vi "Control Screen.vi"() -> ()   [LabVIEW 2016]
uses:
  <vilib>/userdefined/High Color/IMAQdx.ctl
  <vilib>/Utility/file.llb/Read From Spreadsheet File (string).vi
  <vilib>/Utility/file.llb/Write To Spreadsheet File (string).vi
  Library_alfa.lvlib
  <vilib>/vision/driver/NI_Vision_Acquisition_Software.lvlib
  <vilib>/vision/NI_Vision_Development_Module.lvlib
panel:
  in  "Сохранить настройки":bool
  out "индикация видео":T1(plugin-control)
  in  "Область измерения":T2 {"Rotation" format="%.2f"; "Left" scale=0.0..1024.0; "Right" scale=0.0..1280.0}
  in  "Параметры измерения":T3={"Contrast"=40, "Filter width"=4, "Steepness"=2, "Subsampling Ratio"=5, "Show Search Area"=FALSE, "Show Search Lines"=FALSE, "Show Edges Found"=FALSE, "Show Result"=TRUE}
  out "16bit integer":i16
  in  "Уровень бинаризации":T4={"Нижний предел"=128.0, "Верхний предел"=255.0} {"Верхний предел" format="%.2f"; "Нижний предел" format="%.2f"}
  in  "A2":dbl
  in  "A1":dbl
  in  "sp_rol_speed":dbl
  in  "vac":dbl
  out "Номер электрода":string caption="EL NUM"
  out "давл в рессив":string caption="PoR (bar)"
  out "Т газа забор":string caption="ToC (C°)"
  out "WRG":string caption="VoC(torr)"
  out "Давление в камере":string caption="PoC(bar)"
  out "T газа в ролик":string caption="TRG (C°)"
  out "давл блок прив":string caption="PRG (bar)"
  out "T ролик (C°)":string caption="TRB (C°)"
  out "Ист вкл инд":bool caption="WORK"
  out "Давление в плазматроне":string caption="PPG (bar)"
  out "T газ (C°)":string caption="TPG (C°)"
  out "Компрессора диод":bool caption="WORK"
  in  "Компрессора выключить":bool
  in  "Компрессора включить":bool
  out "охлаждение инд":bool caption="WORK"
  in  "Охлаждение выкл":bool
  in  "Охлаждение вкл":bool
  in  "КЗ СТОП":bool
  out "Бункер закрыт":bool caption="WORK"
  in  "Закрыть бункер кн":bool
  in  "Открыть бункер кн":bool
  out "Индикатор положения полки":string
  in  "Бункер на след полку кн":bool
  in  "Аварийный стоп":bool
  in  "Автозапуск регулятора кн":bool
  out "Индикатор автозапуска регулятора":bool
  out "Максимальная подача":string caption="MAX SPEED"
  out "Текущая подача":string caption="SPEED"
  out "Текущий зазор":string caption="DISTANS"
  out "Задание зазора":string caption="SET DISTANS"
  in  "Пересыпное в бол кн":bool
  in  "Пересыпное в малый кн":bool
  out "Пересыпное большой":bool caption="WORK"
  out "Пересыпное малый":bool caption="LOAD"
  out "Бараб V":dbl(knob) caption="ROLLER SPEED" scale=0.0..24000.0
  out "V pl":dbl(knob) caption="VOLTAGE" scale=0.0..100.0
  out "Ток плазматрона":dbl(knob) caption="CURRENT" scale=0.0..2000.0
  out "V бараб":string caption="ROLLER"
  out "Задание част вращ барабанов":string caption="ROLLER SPEED"
  out "вибро 1":string caption="V1 (mm\\s)"
  out "вибро 2":string caption="V1 (mm\\s)"
  out "Ток барабана 2":string caption="S2(A)"
  out "Ток барабана 1":string caption="S1(A)"
  in  "Толкатель поз 2":i32 format="%x"
  in  "Плаз поз 2":i32 format="%x"
  out "плазма рабочее":bool caption="WORK"
  out "положение толк мм":string caption="mm"
  out "Положение плазматрона":string caption="mm"
  out "плазма от заг":bool caption="WORK"
  out "плазма к заг":bool caption="LOAD"
  in  "плазма назад кн":bool
  in  "плазма в раб кн":bool
  out "Толкатель в крайнем":bool caption="WORK"
  out "v_tol":string caption="V (mm\\min)"
  out "v_pl":string caption="V (mm\\min)"
  out "Пол плазматрона":dbl(slide)
  out "Пол толк":dbl(slide) scale=0.0..100.0
  out "Толкатель в рабочем диод":bool caption="WORK"
  out "Толкатель под загрузку диод":bool caption="LOAD"
  in  "Толкатель в рабочее кн":bool
  in  "Толкатель под загрузку кн":bool
  in  "v_pl":i32 format="%x"
  in  "v_tol":i32 format="%x"
  in  "дат вибр 2":i32 format="%x"
  in  "дат вибр1":i32 format="%x"
  in  "ОШИБКА":i32 format="%x"
  in  "T газа в ролик":i32 format="%x"
  in  "давл блок прив":dbl
  in  "Т газа забор":i32 format="%x"
  in  "давл в рессив":dbl
  out "T4 (C°)":string caption="TB2.2 (C°)"
  out "T3 (C°)":string caption="TB2.1 (C°)"
  out "T2 (C°)":string caption="TB1.2 (C°)"
  out "T1 (C°)":string caption="TB1.1 (C°)"
  in  "Подача":i32 format="%x"
  in  "PV":i32 format="%x"
  in  "Roll speed":i32 format="%x"
  in  "P C1":i32 format="%x"
  in  "P plaz":dbl
  in  "ROLLER Speed":dbl
  in  "V плазматр":i32 format="%x"
  in  "Толкатель поз":i32 format="%x"
  in  "Плаз поз":i32 format="%x"
  in  "А плазм":i32 format="%x"
  in  "T GAS":i32 format="%x"
  in  "T ROLLER":i32 format="%x"
  in  "T4":dbl
  in  "T3":i32 format="%x"
  in  "T2":i32 format="%x"
  in  "T1":dbl
  out "Выход":bool caption="WORK"
  in  "Архив":bool
  in  "Газовая система":bool
  in  "Вакуумная система":bool
  in  "Выход":bool
  out "Текущее время":string
  # "DISPENSER"
  # "GAS SYSTEM"
  # "COOLING SYSTEM"
  # "ELECTRODS STORE"
  # "PERFORMANCE PARAMETERS"
  # "PULLEYS"
  # "SP FEED"
  # "PL FEED"
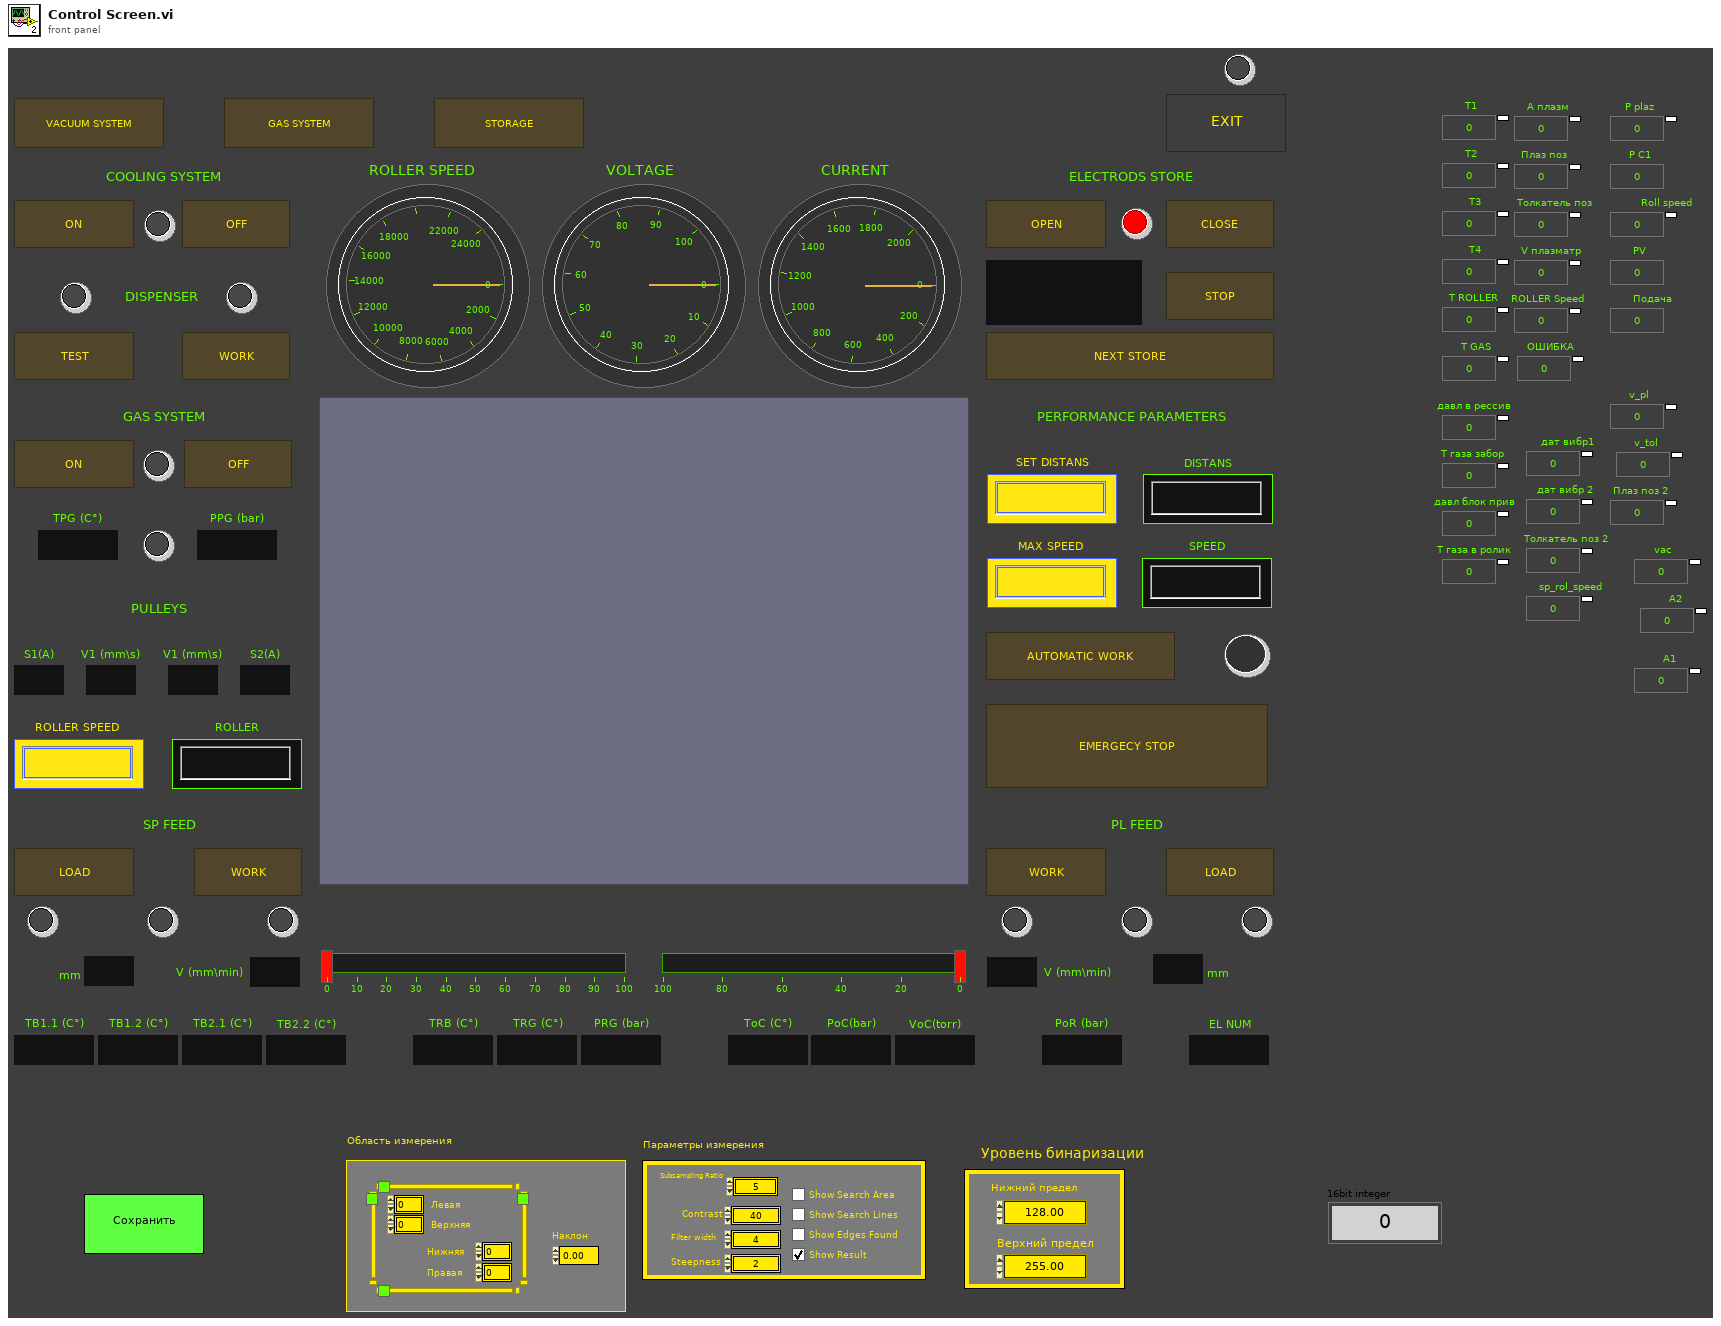
[diagram p1: front panel]
types:
  T1 = typedef "IMAQ Image.ctl" = refnum<image>
  T2 = typedef "IMAQ Rectangle" = cluster{"Left":i32, "Top":i32, "Right":i32, "Bottom":i32, "Rotation":dbl}
  T3 = cluster{"Contrast":i32, "Filter width":i32, "Steepness":i32, "Subsampling Ratio":u32, "Show Search Area":bool, "Show Search Lines":bool, "Show Edges Found":bool, "Show Result":bool}
  T4 = cluster{"Нижний предел":sgl, "Верхний предел":sgl}
  T5 = typedef "Library_alfa.lvlib/IMAQdx.ctl" = refnum<k21>
  T6 = enum16{"open", "replace", "create", "open or create", "replace or create", "replace or create with confirmation"}
  T7 = typedef "Image Type" = u32
  T8 = cluster{i32, i32, i32, u32, "Boolean":bool, "Boolean":bool, "Boolean":bool, "Boolean":bool}
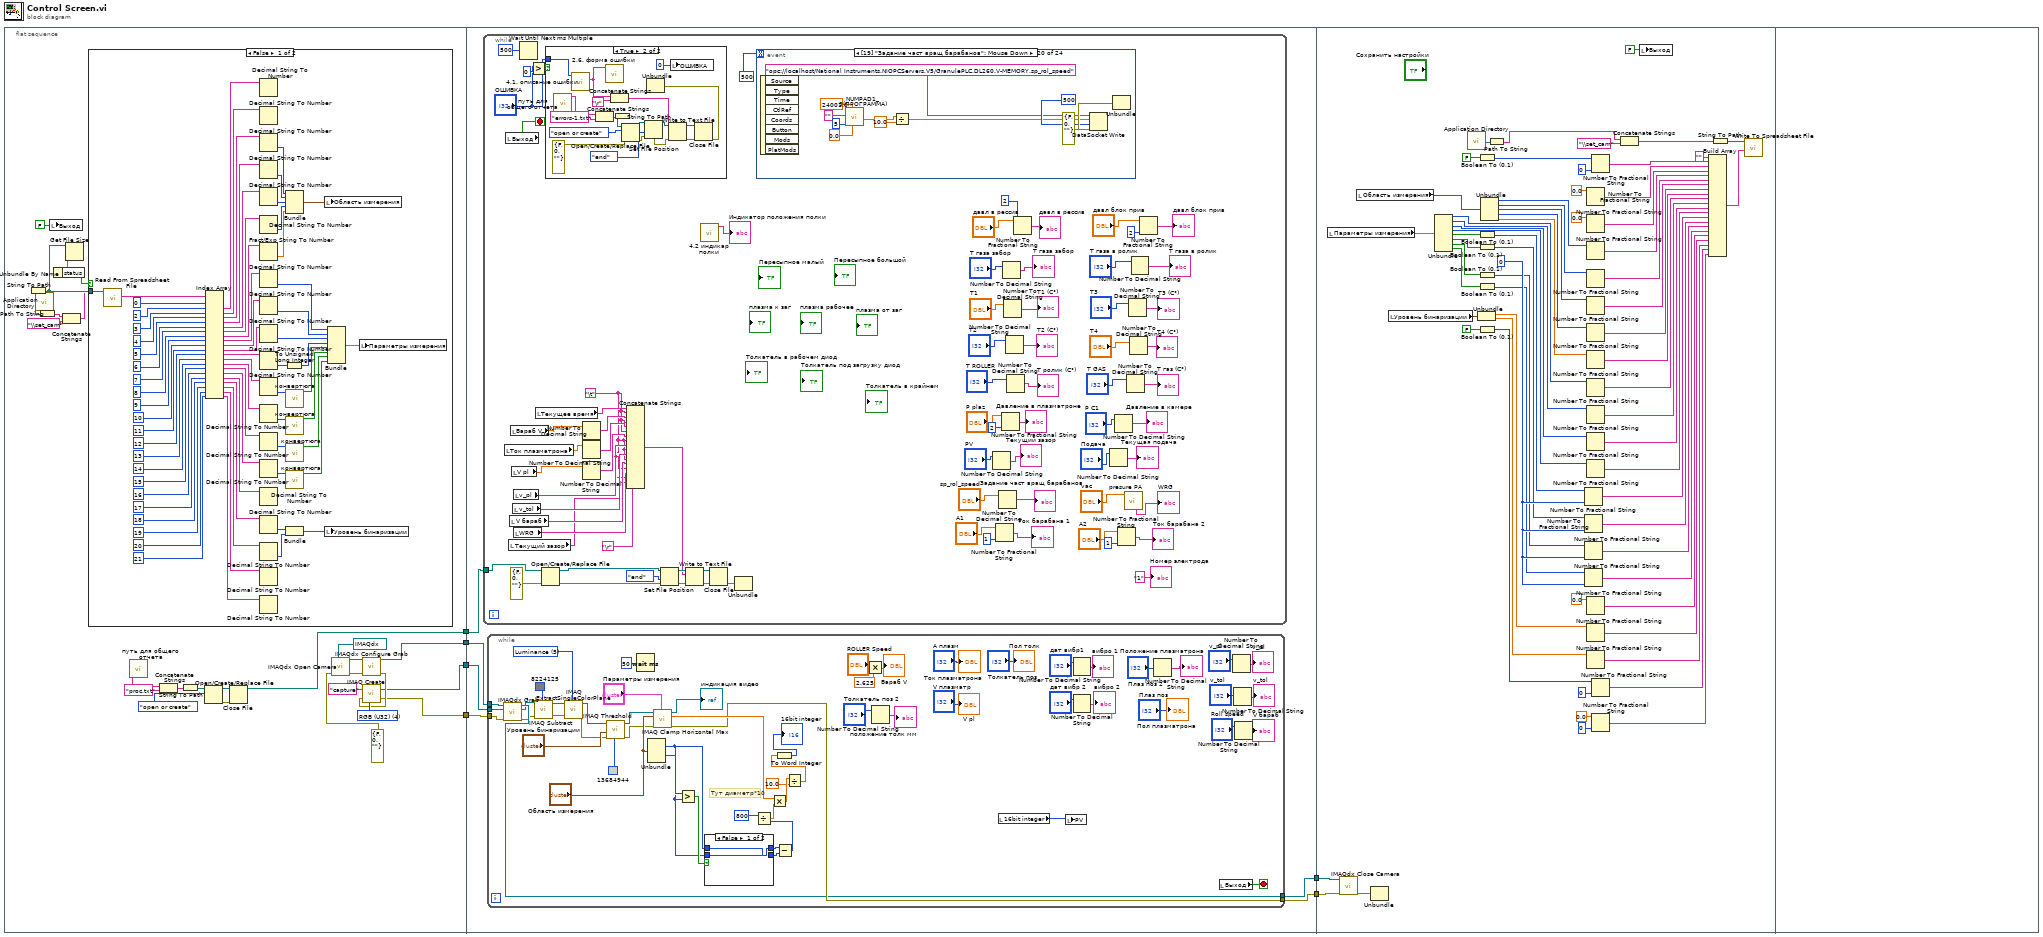
[diagram p0: block diagram]
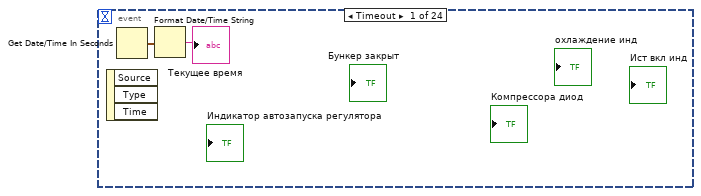
[diagram p5: hidden frame]
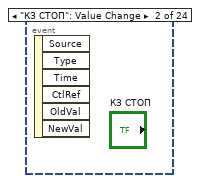
[diagram p6: hidden frame]
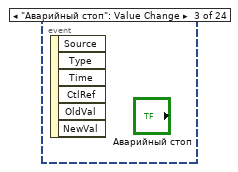
[diagram p7: hidden frame]
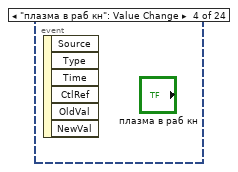
[diagram p8: hidden frame]
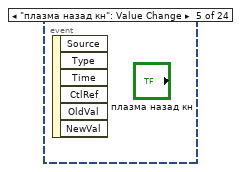
[diagram p9: hidden frame]
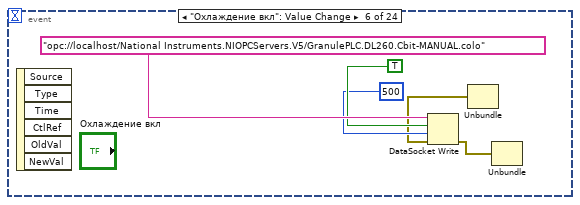
[diagram p10: hidden frame]
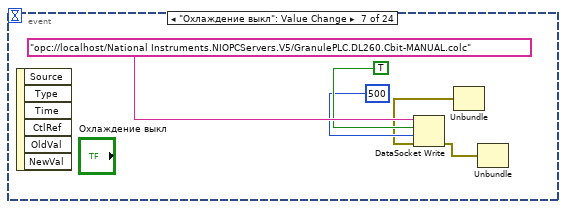
[diagram p11: hidden frame]
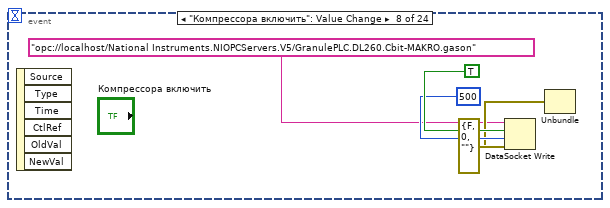
[diagram p12: hidden frame]
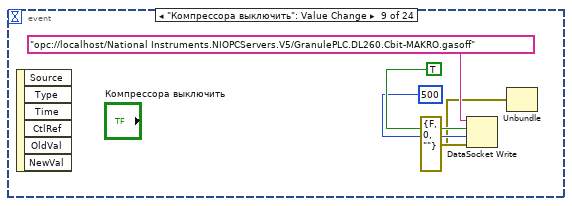
[diagram p13: hidden frame]
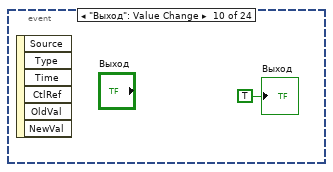
[diagram p14: hidden frame]
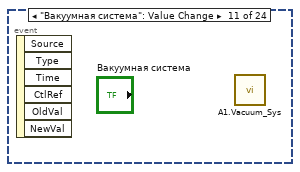
[diagram p15: hidden frame]
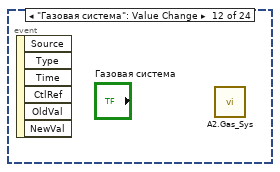
[diagram p16: hidden frame]
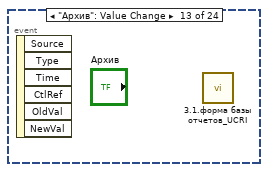
[diagram p17: hidden frame]
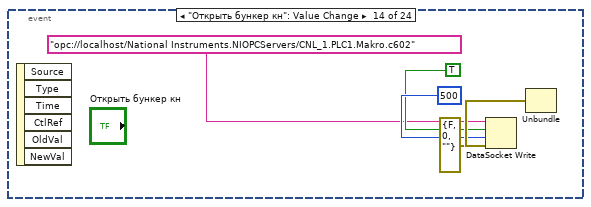
[diagram p18: hidden frame]
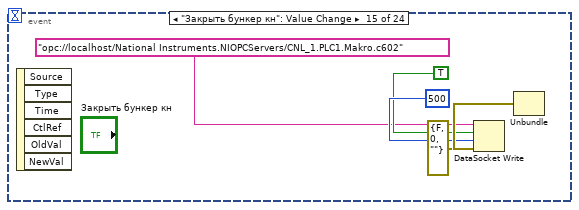
[diagram p19: hidden frame]
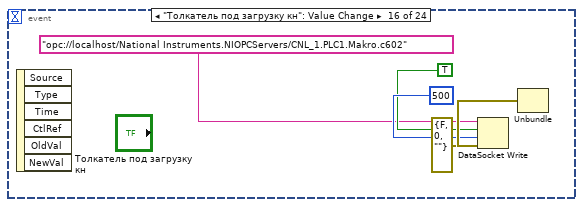
[diagram p20: hidden frame]
diagram:
  n1 = flat-sequence {
    tunnel: [w10] -> w4
    tunnel: [w9] -> w3
    tunnel: [w8] -> w2
    tunnel: [w7] -> w1
    tunnel: [w104] -> w6
    tunnel: [w103] -> w5
    tunnel: w4 -> [w102]
    tunnel: w3 -> [w101]
    tunnel: w2 -> [w100]
    tunnel: w1 -> [w99]
    tunnel: w6 -> [w405]
    tunnel: w5 -> [w404]
    frame #0 {
      w14 = T7 4 items=["Grayscale (U8)", "Grayscale (I16)", "Grayscale (SGL)", "Complex (CSG)", "RGB (U32)", "HSL (U32)", "RGB (U64)", "Grayscale (U16)"] ("Image Type")
      n2 = call <vilib>:"Application Directory.vi"() -> ("Application Directory"=w18:path)
      n3 = Path To String(path=w18) -> (string=w19:string)
      n4 = local write "Выход"(FALSE ("Выход")) -> ()
      n5 = Concatenate Strings(w19, "\\set_cam" ("string")) -> (w21:string)
      n6 = String To Path(string=w21) -> (path=w24:path)
      n7 = Get File Size(file=w24) -> (0:w22:errorcluster)  [unwired: 1 in, 2 out]
      n8 = Unbundle By Name(w22) -> ("status"=w23:bool)
      n9 = case shown="False" w23 {
        tunnel: w24 -> [w98 _]
        frame False {
          n10 = call-poly <vilib>:"Read From Spreadsheet File.vi"("file path (dialog if empty)"=w98) -> ("first row"=w97:string[])  [unwired: 6 in, 4 out]
          n11 = Index Array(array=w97, index #1=0 ("index"), index #2=2 ("index"), index #3=3 ("index"), index #4=4 ("index"), index #5=5 ("index"), index #6=6 ("index"), index #7=7 ("index"), index #8=8 ("index"), index #9=9 ("index"), index #10=10 ("index"), index #11=11 ("index"), index #12=12 ("index"), index #13=13 ("index"), index #14=14 ("index"), index #15=15 ("index"), index #16=16 ("index"), index #17=17 ("index"), index #18=18 ("index"), index #19=19 ("index"), index #20=20 ("index"), index #21=21 ("index")) -> (element #2=w94:string, element #3=w92:string, element #4=w85:string, element #5=w83:string, element #6=w81:string, element #7=w79:string, element #8=w77:string, element #9=w68:string, element #10=w66:string, element #11=w64:string, element #12=w62:string, element #13=w60:string, element #14=w58:string, element #15=w56:string, element #16=w54:string, element #17=w44:string, element #18=w40:string, element #19=w38:string, element #20=w36:string, element #21=w33:string)  [unwired: 1 out]
          n12 = Decimal String To Number(string=w94) -> ()  [unwired: 2 in, 2 out]
          n13 = Decimal String To Number(string=w92) -> ()  [unwired: 2 in, 2 out]
          n14 = Decimal String To Number(string=w85) -> (number=w90:i32)  [unwired: 2 in, 1 out]
          n15 = Decimal String To Number(string=w83) -> (number=w89:i32)  [unwired: 2 in, 1 out]
          n16 = Decimal String To Number(string=w81) -> (number=w88:i32)  [unwired: 2 in, 1 out]
          n17 = Decimal String To Number(string=w79) -> (number=w87:i32)  [unwired: 2 in, 1 out]
          n18 = Fract/Exp String To Number(string=w77) -> (number=w76:dbl)  [unwired: 3 in, 1 out]
          n19 = Decimal String To Number(string=w68) -> (number=w74:i32)  [unwired: 2 in, 1 out]
          n20 = Decimal String To Number(string=w66) -> (number=w73:i32)  [unwired: 2 in, 1 out]
          n21 = Decimal String To Number(string=w64) -> (number=w72:i32)  [unwired: 2 in, 1 out]
          n22 = Decimal String To Number(string=w62) -> (number=w71:i32)  [unwired: 2 in, 1 out]
          n23 = Decimal String To Number(string=w60) -> (number=w53:i32)  [unwired: 2 in, 1 out]
          n24 = Decimal String To Number(string=w58) -> (number=w51:i32)  [unwired: 2 in, 1 out]
          n25 = Decimal String To Number(string=w56) -> (number=w49:i32)  [unwired: 2 in, 1 out]
          n26 = Decimal String To Number(string=w54) -> (number=w47:i32)  [unwired: 2 in, 1 out]
          n27 = Decimal String To Number(string=w44) -> ()  [unwired: 2 in, 2 out]
          n28 = Decimal String To Number(string=w40) -> (number=w39:i32)  [unwired: 2 in, 1 out]
          n29 = Decimal String To Number(string=w38) -> (number=w37:i32)  [unwired: 2 in, 1 out]
          n30 = Decimal String To Number(string=w36) -> ()  [unwired: 2 in, 2 out]
          n31 = Decimal String To Number(string=w33) -> ()  [unwired: 2 in, 2 out]
          n32 = To Unsigned Long Integer(number=w71) -> (unsigned 32bit integer=w70:u32)
          n33 = Bundle(w90, w89, w88, w87, w76) -> (w91:cluster{i32, i32, i32, i32, dbl})  [unwired: 1 in]
          n34 = call "конвертюга.vi"("Numeric"=w53) -> ("Boolean"=w52:bool)  [unwired: 10 in]
          n35 = call "конвертюга.vi"("Numeric"=w51) -> ("Boolean"=w50:bool)  [unwired: 10 in]
          n36 = call "конвертюга.vi"("Numeric"=w49) -> ("Boolean"=w48:bool)  [unwired: 10 in]
          n37 = call "конвертюга.vi"("Numeric"=w47) -> ("Boolean"=w46:bool)  [unwired: 10 in]
          n38 = Bundle(w39, w37) -> (w43:cluster{i32, i32})  [unwired: 1 in]
          n39 = local write "Область измерения"(w91) -> ()
          n40 = local write "Уровень бинаризации"(w43) -> ()
          n41 = Bundle(w74, w73, w72, w70, "Boolean"=w52, "Boolean"=w50, "Boolean"=w48, "Boolean"=w46) -> (w75:T8)  [unwired: 1 in]
          n42 = local write "Параметры измерения"(w75) -> ()
        }
        frame True {
        }
      }
      n43 = call "путь для общего отчета.vi"() -> ("path_out 2"=w28:string)  [unwired: 11 in]
      n44 = Concatenate Strings(w28, "proc.txt") -> (w26:string)
      n45 = String To Path(string=w26) -> (path=w29:path)
      n46 = Open/Create/Replace File(file path (use dialog)=w29, operation (0:open)=T6."open or create") -> (refnum out=w32:refnum<file>, error out=w31:errorcluster)  [unwired: 4 in, 1 out]
      n47 = Close File(refnum=w32, error in=w31) -> (path=w7:path)  [unwired: 1 out]
      n48 = call <vilib>:"IMAQdx Open Camera.vi"("error in"=errorcluster {"status"=FALSE, "code"=0, "source"=""}, "Session In"=T5 "cam3") -> ("error out"=w15:errorcluster, "Session Out"=w12:T5)  [unwired: 8 in]
      n49 = call <vilib>:"IMAQdx Configure Grab.vi"("error in"=w15, "Session In"=w12) -> ("error out"=w11:errorcluster, "Session Out"=w8:T5)  [unwired: 8 in]
      n50 = call "IMAQ Create"("Image Name"="capture", "Image Type"=w14, "error in (no error)"=w11) -> ("New Image"=w10:T1, "error out"=w9:errorcluster)  [unwired: 2 in]
    }
    frame #1 {
      n51 = while {
        tunnel: w99 -> [w181]
        stop <- w237 stop-if-true
        w169 = "\t"
        n52 = local read "Ток плазматрона"() -> (w179:dbl)
        n53 = local read "Выход"() -> (w237:bool)
        n54 = local read "Текущий зазор"() -> (w168:string)
        n55 = local read "V бараб"() -> (w171:string)
        n56 = local read "Бараб V"() -> (w180:dbl)
        n57 = local read "V pl"() -> (w178:dbl)
        n58 = local read "v_tol"() -> (w172:string)
        n59 = local read "v_pl"() -> (w173:string)
        n60 = local read "WRG"() -> (w170:string)
        n61 = Wait Until Next ms Multiple(millisecond multiple=u32 500) -> ()  [unwired: 1 out]
        n62 = Greater?(x="ОШИБКА", y=i16 0) -> (0:w224:bool)
        n63 = local read "Текущее время"() -> (w177:string)
        n64 = Open/Create/Replace File(file path (use dialog)=w181, error in=errorcluster {"status"=FALSE, "code"=0, "source"=""}) -> (refnum out=w190:refnum<file>, error out=w188:errorcluster)  [unwired: 4 in, 1 out]
        n65 = case shown="True" w224 {
          tunnel: "ОШИБКА" -> [_ w241]
          frame False {
          }
          frame True {
            n66 = call "путь для общего отчета.vi"() -> ("path_out 2"=w242:string)  [unwired: 11 in]
            n67 = call "4.1. описание ошибки.vi"("Numeric"=w241) -> ("Полностью"=w240:string)  [unwired: 8 in, 2 out]
            n68 = Concatenate Strings(w242, "errors-1.txt") -> (w256:string)
            n69 = call "2.6. форма ошибки.vi"("Описание ошибки"=w240) -> ()  [unwired: 11 in]
            n70 = Concatenate Strings(w240, "\r") -> (w244:string)
            n71 = String To Path(string=w256) -> (path=w258:path)
            n72 = Open/Create/Replace File(file path (use dialog)=w258, error in=errorcluster {"status"=FALSE, "code"=0, "source"=""}, operation (0:open)=T6."open or create") -> (refnum out=w251:refnum<file>, error out=w253:errorcluster)  [unwired: 3 in, 1 out]
            n73 = Set File Position(refnum=w251, from (0:start)=enum16{"start", "end", "current"}."end", error in=w253) -> (refnum out=w249:refnum<file>, error out=w250:errorcluster)  [unwired: 1 in]
            n74 = Write to Text File(file (use dialog)=w249, text=w244, error in=w250) -> (refnum out=w248:refnum<file>, error out=w247:errorcluster)  [unwired: 1 in, 1 out]
            n75 = local write "ОШИБКА"(i16 0 ("Ошибка1")) -> ()
            n76 = Close File(refnum=w248, error in=w247) -> (error out=w246:errorcluster)  [unwired: 1 out]
            n77 = Unbundle(w246) -> ()  [unwired: 3 out]
          }
        }
        n78 = Number To Decimal String(number=w178) -> (decimal integer string=w174:string)  [unwired: 1 in]
        n79 = Number To Decimal String(number=w180) -> (decimal integer string=w176:string)  [unwired: 1 in]
        n80 = Number To Decimal String(number=w179) -> (decimal integer string=w175:string)  [unwired: 1 in]
        n81 = Concatenate Strings(w177, w169, w176, w169, w175, w169, w174, w169, w173, w169, w172, w169, w171, w169, w170, w169, w168, "\r") -> (w166:string)
        n82 = Set File Position(refnum=w190, from (0:start)=enum16{"start", "end", "current"}."end", error in=w188) -> (refnum out=w187:refnum<file>, error out=w186:errorcluster)  [unwired: 1 in]
        n83 = Write to Text File(file (use dialog)=w187, text=w166, error in=w186) -> (refnum out=w185:refnum<file>, error out=w184:errorcluster)  [unwired: 1 in, 1 out]
        n84 = call "4.2 индикар полки.vi"() -> ("текущее положение"=→"Индикатор положения полки":string)  [unwired: 11 in]
        n85 = Close File(refnum=w185, error in=w184) -> (error out=w183:errorcluster)  [unwired: 1 out]
        n86 = Unbundle(w183) -> ()  [unwired: 3 out]
        n87 = event shown="[19] \"Задание част вращ барабанов\": Mouse Down" {
          selector: _ -> [_ _ _ _ _ _ _ _ _ _ _ _ _ _ _ _ _ _ _ _ _ _ _ _]
          dyn-events: _ -> [_ _ _ _ _ _ _ _ _ _ _ _ _ _ _ _ _ _ _ _ _ _ _ _]
          timeout: 500 -> [_ _ _ _ _ _ _ _ _ _ _ _ _ _ _ _ _ _ _ _ _ _ _ _]
          event Timeout {
            n88 = event-data() -> ()  [unwired: 1 in, 3 out]
            n89 = Get Date/Time In Seconds() -> (seconds since 1Jan1904=w260:timestamp)
            n90 = Format Date/Time String(seconds (now)=w260) -> (date/time string=→"Текущее время":string)  [unwired: 2 in]
          }
          event "КЗ СТОП": Value Change {
            n91 = event-data() -> ()  [unwired: 1 in, 6 out]
          }
          event "Аварийный стоп": Value Change {
            n92 = event-data() -> ()  [unwired: 1 in, 6 out]
          }
          event "плазма в раб кн": Value Change {
            n93 = event-data() -> ()  [unwired: 1 in, 6 out]
          }
          event "плазма назад кн": Value Change {
            n94 = event-data() -> ()  [unwired: 1 in, 6 out]
          }
          event "Охлаждение вкл": Value Change {
            n95 = event-data() -> ()  [unwired: 1 in, 6 out]
            n96 = DataSocket Write(9:500 ("ms timeout (0)"), 10:TRUE, 11:"opc://localhost/National Instruments.NIOPCServers.V5/GranulePLC.DL260.Cbit-MANUAL.colo" ("connection in")) -> (0:w261:errorcluster)  [unwired: 1 in, 2 out]
            n97 = Unbundle(w261) -> ()  [unwired: 3 out]
            n98 = Unbundle(w261) -> ()  [unwired: 3 out]
          }
          event "Охлаждение выкл": Value Change {
            n99 = event-data() -> ()  [unwired: 1 in, 6 out]
            n100 = DataSocket Write(9:500 ("ms timeout (0)"), 10:TRUE, 11:"opc://localhost/National Instruments.NIOPCServers.V5/GranulePLC.DL260.Cbit-MANUAL.colc" ("connection in")) -> (0:w265:errorcluster)  [unwired: 1 in, 2 out]
            n101 = Unbundle(w265) -> ()  [unwired: 3 out]
            n102 = Unbundle(w265) -> ()  [unwired: 3 out]
          }
          event "Компрессора включить": Value Change {
            n103 = event-data() -> ()  [unwired: 1 in, 6 out]
            n104 = DataSocket Write(8:errorcluster {"status"=FALSE, "code"=0, "source"=""} ("error in (no error)"), 9:500 ("ms timeout (0)"), 10:TRUE, 11:"opc://localhost/National Instruments.NIOPCServers.V5/GranulePLC.DL260.Cbit-MAKRO.gason" ("connection in")) -> (0:w270:errorcluster)  [unwired: 2 out]
            n105 = Unbundle(w270) -> ()  [unwired: 3 out]
          }
          event "Компрессора выключить": Value Change {
            n106 = event-data() -> ()  [unwired: 1 in, 6 out]
            n107 = DataSocket Write(8:errorcluster {"status"=FALSE, "code"=0, "source"=""} ("error in (no error)"), 9:500 ("ms timeout (0)"), 10:TRUE, 11:"opc://localhost/National Instruments.NIOPCServers.V5/GranulePLC.DL260.Cbit-MAKRO.gasoff" ("connection in")) -> (0:w274:errorcluster)  [unwired: 2 out]
            n108 = Unbundle(w274) -> ()  [unwired: 3 out]
          }
          event "Выход": Value Change {
            n109 = event-data() -> ()  [unwired: 1 in, 6 out]
            "Выход" <- TRUE ("Выход")
          }
          event "Вакуумная система": Value Change {
            n110 = event-data() -> ()  [unwired: 1 in, 6 out]
            n111 = call "A1.Vacuum_Sys.vi"() -> ()  [unwired: 12 in]
          }
          event "Газовая система": Value Change {
            n112 = event-data() -> ()  [unwired: 1 in, 6 out]
            n113 = call "A2.Gas_Sys.vi"() -> ()  [unwired: 12 in]
          }
          event "Архив": Value Change {
            n114 = event-data() -> ()  [unwired: 1 in, 6 out]
            n115 = call "3.1.форма базы отчетов_UCRI.vi"() -> ()  [unwired: 12 in]
          }
          event "Открыть бункер кн": Value Change {
            n116 = event-data() -> ()  [unwired: 1 in, 6 out]
            n117 = DataSocket Write(8:errorcluster {"status"=FALSE, "code"=0, "source"=""} ("error in (no error)"), 9:500 ("ms timeout (0)"), 10:TRUE, 11:"opc://localhost/National Instruments.NIOPCServers/CNL_1.PLC1.Makro.c602" ("connection in")) -> (0:w284:errorcluster)  [unwired: 2 out]
            n118 = Unbundle(w284) -> ()  [unwired: 3 out]
          }
          event "Закрыть бункер кн": Value Change {
            n119 = event-data() -> ()  [unwired: 1 in, 6 out]
            n120 = DataSocket Write(8:errorcluster {"status"=FALSE, "code"=0, "source"=""} ("error in (no error)"), 9:500 ("ms timeout (0)"), 10:TRUE, 11:"opc://localhost/National Instruments.NIOPCServers/CNL_1.PLC1.Makro.c602" ("connection in")) -> (0:w289:errorcluster)  [unwired: 2 out]
            n121 = Unbundle(w289) -> ()  [unwired: 3 out]
          }
          event "Толкатель под загрузку кн": Value Change {
            n122 = event-data() -> ()  [unwired: 1 in, 6 out]
            n123 = DataSocket Write(8:errorcluster {"status"=FALSE, "code"=0, "source"=""} ("error in (no error)"), 9:500 ("ms timeout (0)"), 10:TRUE, 11:"opc://localhost/National Instruments.NIOPCServers/CNL_1.PLC1.Makro.c602" ("connection in")) -> (0:w294:errorcluster)  [unwired: 2 out]
            n124 = Unbundle(w294) -> ()  [unwired: 3 out]
          }
          event "Толкатель в рабочее кн": Value Change {
            n125 = event-data() -> ()  [unwired: 1 in, 6 out]
            n126 = DataSocket Write(8:errorcluster {"status"=FALSE, "code"=0, "source"=""} ("error in (no error)"), 9:500 ("ms timeout (0)"), 10:TRUE, 11:"opc://localhost/National Instruments.NIOPCServers/CNL_1.PLC1.Makro.c602" ("connection in")) -> (0:w295:errorcluster)  [unwired: 2 out]
            n127 = Unbundle(w295) -> ()  [unwired: 3 out]
          }
          event "Бункер на след полку кн": Value Change {
            n128 = event-data() -> ()  [unwired: 1 in, 6 out]
            n129 = DataSocket Write(8:errorcluster {"status"=FALSE, "code"=0, "source"=""} ("error in (no error)"), 9:500 ("ms timeout (0)"), 10:TRUE, 11:"opc://localhost/National Instruments.NIOPCServers/CNL_1.PLC1.Makro.c602" ("connection in")) -> (0:w304:errorcluster)  [unwired: 2 out]
            n130 = Unbundle(w304) -> ()  [unwired: 3 out]
          }
          event "Автозапуск регулятора кн": Value Change {
            n131 = event-data() -> ()  [unwired: 1 in, 6 out]
            n132 = DataSocket Write(8:errorcluster {"status"=FALSE, "code"=0, "source"=""} ("error in (no error)"), 9:500 ("ms timeout (0)"), 10:TRUE, 11:"opc://localhost/National Instruments.NIOPCServers.V5/GranulePLC.DL260.Cbit-MAKRO.rid_run" ("connection in")) -> (0:w309:errorcluster)  [unwired: 2 out]
            n133 = Unbundle(w309) -> ()  [unwired: 3 out]
          }
          event "Задание част вращ барабанов": Mouse Down {
            n134 = event-data() -> ()  [unwired: 1 in, 8 out]
            n135 = call "NUMPAD1_9(ПРОГРАММА).vi"("МИНИМАЛЬНОЕ ЗНАЧЕНИЕ"=0.0, "МАКСИМАЛЬНОЕ ЗНАЧЕНИЕ"=24001.0, "ДЛИННА СЛОВА"=i8 5, "ТЕКУЩЕЕ ЗНАЧЕНИЕ"="") -> ("exit"=w311:dbl)  [unwired: 6 in, 1 out]
            n136 = Divide(x=w311, y=10.0) -> (x/y=w312:dbl)
            n137 = DataSocket Write(8:errorcluster {"status"=FALSE, "code"=0, "source"=""} ("error in (no error)"), 9:500 ("ms timeout (0)"), 10:w312, 11:"opc://localhost/National Instruments.NIOPCServers.V5/GranulePLC.DL260.V-MEMORY.sp_rol_speed" ("connection in")) -> (0:w320:errorcluster)  [unwired: 2 out]
            n138 = Unbundle(w320) -> ()  [unwired: 3 out]
          }
          event "Максимальная подача": Mouse Down {
            n139 = event-data() -> ()  [unwired: 1 in, 8 out]
            n140 = DataSocket Write(8:errorcluster {"status"=FALSE, "code"=0, "source"=""} ("error in (no error)"), 9:500 ("ms timeout (0)"), 10:TRUE, 11:"opc://localhost/National Instruments.NIOPCServers/CNL_1.PLC1.Makro.c602" ("connection in")) -> (0:w325:errorcluster)  [unwired: 2 out]
            n141 = Unbundle(w325) -> ()  [unwired: 3 out]
          }
          event "Пересыпное в малый кн": Value Change {
            n142 = event-data() -> ()  [unwired: 1 in, 6 out]
            n143 = DataSocket Write(8:errorcluster {"status"=FALSE, "code"=0, "source"=""} ("error in (no error)"), 9:500 ("ms timeout (0)"), 10:TRUE, 11:"opc://localhost/National Instruments.NIOPCServers.V5/GranulePLC.DL260.Cbit-MANUAL.ptm" ("connection in")) -> (0:w330:errorcluster)  [unwired: 2 out]
            n144 = Unbundle(w330) -> ()  [unwired: 3 out]
          }
          event "Пересыпное в бол кн": Value Change {
            n145 = event-data() -> ()  [unwired: 1 in, 6 out]
            n146 = DataSocket Write(8:errorcluster {"status"=FALSE, "code"=0, "source"=""} ("error in (no error)"), 9:500 ("ms timeout (0)"), 10:TRUE, 11:"opc://localhost/National Instruments.NIOPCServers.V5/GranulePLC.DL260.Cbit-MANUAL.ptb" ("connection in")) -> (0:w335:errorcluster)  [unwired: 2 out]
            n147 = Unbundle(w335) -> ()  [unwired: 3 out]
          }
          event "Задание зазора": Mouse Down {
            n148 = event-data() -> ()  [unwired: 1 in, 8 out]
            n149 = DataSocket Write(8:errorcluster {"status"=FALSE, "code"=0, "source"=""} ("error in (no error)"), 9:500 ("ms timeout (0)"), 10:TRUE, 11:"opc://localhost/National Instruments.NIOPCServers/CNL_1.PLC1.Makro.c602" ("connection in")) -> (0:w340:errorcluster)  [unwired: 2 out]
            n150 = Unbundle(w340) -> ()  [unwired: 3 out]
          }
        }
        n151 = Number To Decimal String(number="PV") -> (decimal integer string=→"Текущий зазор":string)  [unwired: 1 in]
        n152 = Number To Fractional String(number="A1", precision (6)=i16 1) -> (F-format string=→"Ток барабана 1":string)  [unwired: 2 in]
        n153 = Number To Decimal String(number="sp_rol_speed") -> (decimal integer string=→"Задание част вращ барабанов":string)  [unwired: 1 in]
        n154 = Number To Fractional String(number="P plaz", precision (6)=i16 2) -> (F-format string=→"Давление в плазматроне":string)  [unwired: 2 in]
        n155 = Number To Decimal String(number="Т газа забор") -> (decimal integer string=→"Т газа забор":string)  [unwired: 1 in]
        n156 = Number To Decimal String(number="T1") -> (decimal integer string=→"T1 (C°)":string)  [unwired: 1 in]
        n157 = Number To Decimal String(number="T2") -> (decimal integer string=→"T2 (C°)":string)  [unwired: 1 in]
        n158 = Number To Decimal String(number="T ROLLER") -> (decimal integer string=→"T ролик (C°)":string)  [unwired: 1 in]
        n159 = Number To Fractional String(number="давл в рессив", precision (6)=i16 2) -> (F-format string=→"давл в рессив":string)  [unwired: 2 in]
        n160 = Number To Decimal String(number="Подача") -> (decimal integer string=→"Текущая подача":string)  [unwired: 1 in]
        n161 = Number To Decimal String(number="P C1") -> (decimal integer string=→"Давление в камере":string)  [unwired: 1 in]
        n162 = Number To Fractional String(number="A2", precision (6)=i16 1) -> (F-format string=→"Ток барабана 2":string)  [unwired: 2 in]
        n163 = call "presure PA.vi"("Volte"="vac") -> ("presure String 2"=→"WRG":string)  [unwired: 7 in, 3 out]
        n164 = Number To Decimal String(number="T GAS") -> (decimal integer string=→"T газ (C°)":string)  [unwired: 1 in]
        n165 = Number To Decimal String(number="T3") -> (decimal integer string=→"T3 (C°)":string)  [unwired: 1 in]
        n166 = Number To Decimal String(number="T4") -> (decimal integer string=→"T4 (C°)":string)  [unwired: 1 in]
        n167 = Number To Decimal String(number="T газа в ролик") -> (decimal integer string=→"T газа в ролик":string)  [unwired: 1 in]
        n168 = Number To Fractional String(number="давл блок прив", precision (6)=i16 2) -> (F-format string=→"давл блок прив":string)  [unwired: 2 in]
        "Номер электрода" <- "1" ("Номер электрода")
      }
      n169 = while {
        tunnel: w101 -> [w132]
        tunnel: [w134] -> w104
        tunnel: [w136] -> w103
        tunnel: w102 -> [w108]
        tunnel: w100 -> [w107]
        stop <- w161 stop-if-true
        w130 = 5 items=["Red", "Green", "Blue", "Hue", "Saturation", "Luminance", "Value", "Intensity"] ("Color Plane")
        # "Тут диаметр*10"
        n170 = call <vilib>:"IMAQdx Grab.vi"("error in"=w132, "Image In"=w108, "Session In"=w107) -> ("error out"=w133:errorcluster, "Image Out"=w105:T1, "Session Out"=w134:T5)  [unwired: 5 in, 1 out]
        n171 = call "IMAQ Subtract"("Image Src A"=w105, "Constant"=u32 8224125 ("Калибровка"), "error in (no error)"=w133) -> ("Image Dst Out"=w158:T1, "error out"=w144:errorcluster)  [unwired: 4 in]
        n172 = call "IMAQ ExtractSingleColorPlane"("Color Plane"=w130, "error in (no error)"=w144, "Image Src"=w158) -> ("error out"=w143:errorcluster, "Image Dst Out"=w145:T1)  [unwired: 7 in]
        n173 = call "IMAQ Threshold"("Replace Value"=u32 13684944 ("Рабочий цвет"), "error in (no error)"=w143, "Range"="Уровень бинаризации", "Image Src"=w145) -> ("error out"=w141:errorcluster, "Image Dst Out"=w142:T1)  [unwired: 2 in, 4 out]
        n174 = Wait (ms)(milliseconds to wait=u32 50) -> ()  [unwired: 1 out]
        n175 = Unbundle("Область измерения") -> ("Top"=w149:i32, "Bottom"=w148:i32)  [unwired: 3 out]
        n176 = call "IMAQ Clamp Horizontal Max"("Settings"="Параметры измерения", "error in (no error)"=w141, "Rectangle"="Область измерения", "Image"=w142) -> ("error out"=w136:errorcluster, "Distance"=w157:sgl, "Image Out"=→"индикация видео":T1)  [unwired: 3 in, 2 out]
        n177 = Greater?(x=w149, y=w148) -> (0:w151:bool)
        n178 = case shown="False" w151 {
          tunnel: [w163 w165] -> w150
          tunnel: w149 -> [w162 w165]
          tunnel: w148 -> [w163 w164]
          tunnel: [w162 w164] -> w147
          frame False {
          }
          frame True {
          }
        }
        n179 = Subtract(x=w150, y=w147) -> (x-y=w153:i32)
        n180 = Divide(x=800, y=w153) -> (x/y=w152:dbl)
        n181 = Multiply(x=w157, y=w152) -> (x*y=w156:dbl)
        n182 = Divide(x=w156, y=10.0) -> (x/y=w139:dbl)
        n183 = To Word Integer(number=w139) -> (16bit integer=→"16bit integer":i16)
        n184 = Multiply(x="ROLLER Speed", y=2.625) -> (x*y=→"Бараб V":dbl)
        n185 = Number To Decimal String(number="Толкатель поз 2") -> (decimal integer string=→"положение толк мм":string)  [unwired: 1 in]
        n186 = local read "16bit integer"() -> (w106:i16)
        n187 = local write "PV"(w106) -> ()
        n188 = Number To Decimal String(number="дат вибр1") -> (decimal integer string=→"вибро 1":string)  [unwired: 1 in]
        n189 = Number To Decimal String(number="дат вибр 2") -> (decimal integer string=→"вибро 2":string)  [unwired: 1 in]
        n190 = Number To Decimal String(number="Плаз поз 2") -> (decimal integer string=→"Положение плазматрона":string)  [unwired: 1 in]
        n191 = local read "Выход"() -> (w161:bool)
        n192 = Number To Decimal String(number="v_pl") -> (decimal integer string=→"v_pl":string)  [unwired: 1 in]
        n193 = Number To Decimal String(number="v_tol") -> (decimal integer string=→"v_tol":string)  [unwired: 1 in]
        n194 = Number To Decimal String(number="Roll speed") -> (decimal integer string=→"V бараб":string)  [unwired: 1 in]
        "Пол плазматрона" <- "Плаз поз"
        "Ток плазматрона" <- "А плазм"
        "V pl" <- "V плазматр"
        "Пол толк" <- "Толкатель поз"
      }
    }
    frame #2 {
      w385 = i16 0 ("precision (6)")
      n195 = local read "Параметры измерения"() -> (w348:T3)
      n196 = call <vilib>:"IMAQdx Close Camera.vi"("error in"=w404, "Session In"=w405) -> ("error out"=w403:errorcluster)  [unwired: 9 in]
      n197 = local read "Область измерения"() -> (w341:T2)
      n198 = Unbundle(w403) -> ()  [unwired: 3 out]
      n199 = local read "Уровень бинаризации"() -> (w361:T4)
      n200 = Unbundle(w348) -> ("Contrast"=w349:i32, "Filter width"=w350:i32, "Steepness"=w351:i32, "Subsampling Ratio"=w352:u32, "Show Search Area"=w353:bool, "Show Search Lines"=w354:bool, "Show Edges Found"=w355:bool, "Show Result"=w356:bool)
      n201 = call <vilib>:"Application Directory.vi"() -> ("Application Directory"=w389:path)
      n202 = Unbundle(w361) -> ("Нижний предел"=w362:sgl, "Верхний предел"=w363:sgl)
      n203 = Boolean To (0,1)(Boolean=FALSE) -> (0, 1=w342:i16)
      n204 = Boolean To (0,1)(Boolean=w353) -> (0, 1=w357:i16)
      n205 = Boolean To (0,1)(Boolean=w354) -> (0, 1=w358:i16)
      n206 = Boolean To (0,1)(Boolean=w355) -> (0, 1=w359:i16)
      n207 = Boolean To (0,1)(Boolean=w356) -> (0, 1=w360:i16)
      n208 = Boolean To (0,1)(Boolean=FALSE) -> (0, 1=w383:i16)
      n209 = Unbundle(w341) -> ("Left"=w343:i32, "Top"=w344:i32, "Right"=w345:i32, "Bottom"=w346:i32, "Rotation"=w347:dbl)
      n210 = Path To String(path=w389) -> (string=w390:string)
      n211 = Number To Fractional String(number=w357, precision (6)=w385) -> (F-format string=w376:string)  [unwired: 2 in]
      n212 = Number To Fractional String(number=w358, precision (6)=w385) -> (F-format string=w377:string)  [unwired: 2 in]
      n213 = Number To Fractional String(number=w359, precision (6)=w385) -> (F-format string=w378:string)  [unwired: 2 in]
      n214 = Number To Fractional String(number=w360, precision (6)=w385) -> (F-format string=w379:string)  [unwired: 2 in]
      n215 = Number To Fractional String(number=0.0) -> (F-format string=w365:string)  [unwired: 3 in]
      n216 = Number To Fractional String(number=0.0) -> (F-format string=w366:string)  [unwired: 3 in]
      n217 = Number To Fractional String(number=w343) -> (F-format string=w367:string)  [unwired: 3 in]
      n218 = Number To Fractional String(number=w344) -> (F-format string=w368:string)  [unwired: 3 in]
      n219 = Number To Fractional String(number=w345) -> (F-format string=w369:string)  [unwired: 3 in]
      n220 = Number To Fractional String(number=w346) -> (F-format string=w370:string)  [unwired: 3 in]
      n221 = Number To Fractional String(number=w347) -> (F-format string=w371:string)  [unwired: 3 in]
      n222 = Number To Fractional String(number=w349) -> (F-format string=w372:string)  [unwired: 3 in]
      n223 = Number To Fractional String(number=w350) -> (F-format string=w373:string)  [unwired: 3 in]
      n224 = Number To Fractional String(number=w351) -> (F-format string=w374:string)  [unwired: 3 in]
      n225 = Number To Fractional String(number=w352) -> (F-format string=w375:string)  [unwired: 3 in]
      n226 = Number To Fractional String(number=0.0) -> (F-format string=w380:string)  [unwired: 3 in]
      n227 = Number To Fractional String(number=w362) -> (F-format string=w381:string)  [unwired: 3 in]
      n228 = Number To Fractional String(number=w363) -> (F-format string=w382:string)  [unwired: 3 in]
      n229 = Number To Fractional String(number=w342, precision (6)=i16 0) -> (F-format string=w364:string)  [unwired: 2 in]
      n230 = Number To Fractional String(number=w383, precision (6)=i16 0) -> (F-format string=w384:string)  [unwired: 2 in]
      n231 = Number To Fractional String(number=0.0, precision (6)=i16 0) -> (F-format string=w395:string)  [unwired: 2 in]
      n232 = Concatenate Strings(w390, "\\set_cam" ("string")) -> (w392:string)
      n233 = local write "Выход"(FALSE ("Выход")) -> ()
      n234 = Build Array("" ("element"), w364, w365, w366, w367, w368, w369, w370, w371, w372, w373, w374, w375, w376, w377, w378, w379, w380, w381, w382, w384, w395) -> (w388:string[])
      n235 = String To Path(string=w392) -> (path=w393:path)
      n236 = call-poly <vilib>:"Write To Spreadsheet File.vi"("1D data"=w388, "file path (dialog if empty)"=w393) -> ()  [unwired: 6 in, 1 out]
    }
    frame #3 {
    }
  }
